vi "find_repeat_parameters_2.vi"(8 "error in (no error)":errorcluster, 11 "String In":string="[SENSe[1]]|SENSe2:SWEep[1]|2|3|4:AUTO:REF1|REF2\n<numeric_value>") -> (0 "error out":errorcluster, 3 "String Out":string="[SENSe[1]]|SENSe2:SWEep[1]|2|3|4:AUTO:REF{<n>}\n<numeric_value>")   [LabVIEW 2018]
uses:
  <vilib>/regexp/Match Regular Expression.xnode
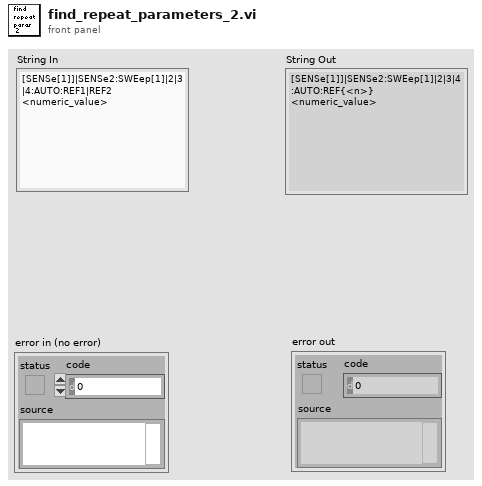
[diagram p1: front panel]
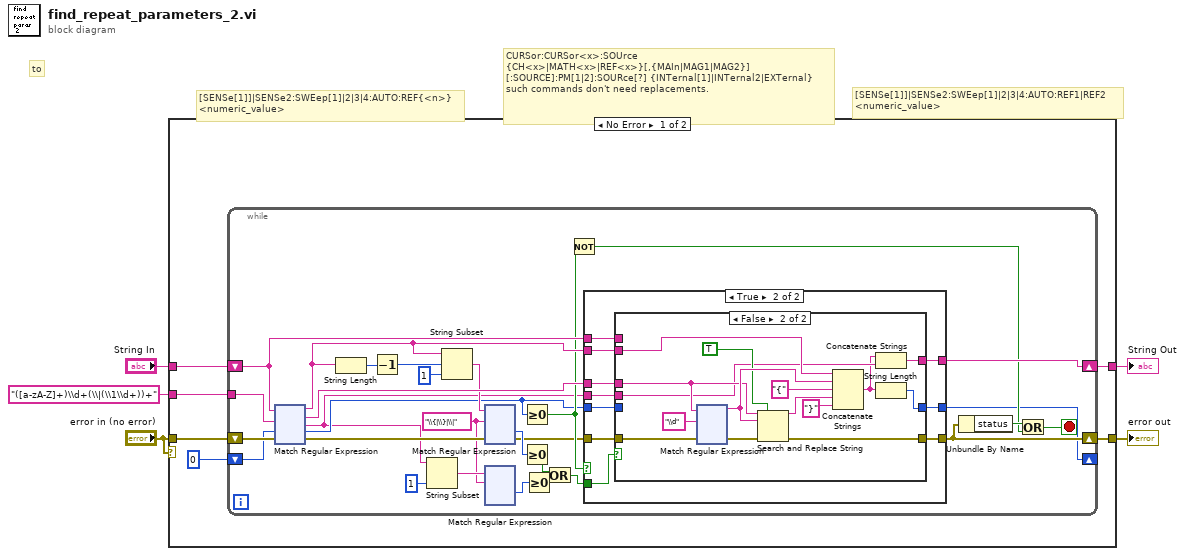
[diagram p0: block diagram]
diagram:
  # "CURSor:CURSor<x>:SOUrce \n{CH<x>|MATH<x>|REF<x>}[,{MAIn|MAG1|MAG2}]\n[:SOURCE]:PM[1|2]:SOURce[?] {INTernal[1]|INTernal2|EXTernal}\nsuch commands don't need replacements."
  # "to"
  # "[SENSe[1]]|SENSe2:SWEep[1]|2|3|4:AUTO:REF{<n>}\n<numeric_value>"
  # "[SENSe[1]]|SENSe2:SWEep[1]|2|3|4:AUTO:REF1|REF2\n<numeric_value>"
  n1 = case shown="No Error" "error in (no error)" {
    tunnel: "([a-zA-Z]+)\\d+(\\|(\\1\\d+))+" ("regular expression") -> [w11 _]
    tunnel: "String In" -> [w8 w517]
    tunnel: [w10 w517] -> w3
    tunnel: "error in (no error)" -> [w7 w516]
    tunnel: [w9 w516] -> w2
    frame No Error {
      n2 = while {
        tunnel: w11 -> [w40]
        shift-right: [w38] -> w10
        shift-left: w8 -> [w31]
        shift-right: [w22] -> w9
        shift-left: w7 -> [w30]
        shift-right: [w21] -> _
        shift-left: 0 ("offset (0)") -> [w25]
        stop <- w28 stop-if-true
        w16 = "\\{|\\}|\\|" ("regular expression")
        n3 = xnode "Match Regular Expression"("input string"=w31, "regular expression"=w40, "offset (0)"=w25, "error in"=w30) -> ("before match"=w35:string, "whole match"=w39:string, "after match"=w18:string, "offset past match"=w20:i32, "error out"=w24:errorcluster)  [unwired: 2 out]
        n4 = String Length(string=w35) -> (length=w36:i32)
        n5 = Decrement(x=w36) -> (x-1=w37:i32)
        n6 = String Subset(string=w18, length (rest)=1 ("length (rest)")) -> (substring=w17:string)  [unwired: 1 out]
        n7 = String Subset(string=w35, offset (0)=w37, length (rest)=1 ("length (rest)")) -> (substring=w33:string)
        n8 = xnode "Match Regular Expression"("input string"=w33, "regular expression"=w16, "error in"=w24) -> ("offset past match"=w32:i32, "error out"=w23:errorcluster)  [unwired: 1 in, 5 out]
        n9 = xnode "Match Regular Expression"("input string"=w17, "regular expression"=w16) -> ("offset past match"=w15:i32)  [unwired: 2 in, 6 out]
        n10 = Greater Or Equal To 0?(x=w20) -> (x >= 0?=w26:bool)
        n11 = Greater Or Equal To 0?(x=w32) -> (x >= 0?=w14:bool)
        n12 = Greater Or Equal To 0?(x=w15) -> (x >= 0?=w13:bool)
        n13 = Or(x=w14, y=w13) -> (x .or. y?=w12:bool)
        n14 = Not(x=w26) -> (.not. x?=w27:bool)
        n15 = case shown="True" w26 {
          tunnel: w39 -> [_ w164]
          tunnel: [w154 w163] -> w38
          tunnel: w35 -> [_ w162]
          tunnel: w18 -> [_ w161]
          tunnel: w31 -> [w154 w160]
          tunnel: w23 -> [w153 w159]
          tunnel: [w153 w158] -> w22
          tunnel: [w152 w157] -> w21
          tunnel: w20 -> [w152 w156]
          tunnel: w12 -> [_ w155]
          frame False {
          }
          frame True {
            n16 = case shown="False" w155 {
              tunnel: w164 -> [_ w179]
              tunnel: [w167 w168] -> w163
              tunnel: w162 -> [_ w182]
              tunnel: w161 -> [_ w171]
              tunnel: w160 -> [w167 _]
              tunnel: w159 -> [w166 w174]
              tunnel: [w166 w172] -> w158
              tunnel: [w165 w169] -> w157
              tunnel: w156 -> [w165 _]
              frame True {
              }
              frame False {
                n17 = xnode "Match Regular Expression"("input string"=w179, "regular expression"="\\d", "error in"=w174) -> ("before match"=w180:string, "error out"=w173:errorcluster)  [unwired: 1 in, 5 out]
                n18 = Search and Replace String(replace all?=TRUE ("replace all? (F)"), input string=w179, search string=w180, error in=w173) -> (result string=w177:string, error out=w172:errorcluster)  [unwired: 6 out]
                n19 = Concatenate Strings(w182, w180, "{" ("string"), w177, "}" ("string")) -> (w170:string)
                n20 = Concatenate Strings(w170, w171) -> (w168:string)
                n21 = String Length(string=w170) -> (length=w169:i32)
              }
            }
          }
        }
        n22 = Unbundle By Name(w22) -> ("status"=w29:bool)
        n23 = Or(x=w29, y=w27) -> (x .or. y?=w28:bool)
      }
    }
    frame Error {
    }
  }
  "String Out" <- w3
  "error out" <- w2
